vi "TestQTMCommander.vi"() -> ()   [LabVIEW 2017]
uses:
  Globals/QualisysInstruction.vi
panel:
  in  "StopCapture":bool
  in  "SendTrig":bool
  in  "stop":bool
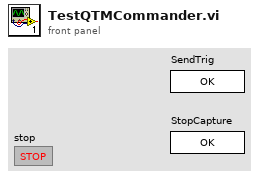
[diagram p1: front panel]
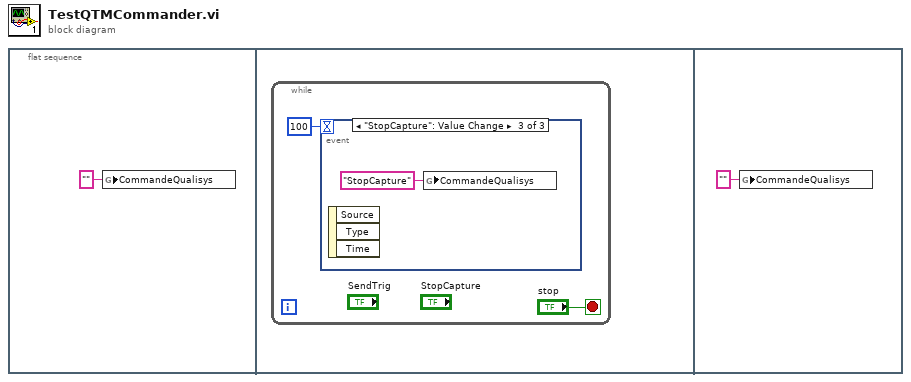
[diagram p0: block diagram]
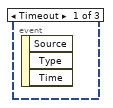
[diagram p2: hidden frame]
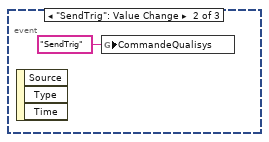
[diagram p3: hidden frame]
diagram:
  n1 = flat-sequence {
    frame #0 {
      n2 = global write "QualisysInstruction.vi" "CommandeQualisys"("" ("CommandeQualisys")) -> ()
    }
    frame #1 {
      n3 = while {
        stop <- "stop" stop-if-true
        n4 = event shown="[2] \"StopCapture\": Value Change" {
          selector: _ -> [_ _ _]
          dyn-events: _ -> [_ _ _]
          timeout: 100 -> [_ _ _]
          event Timeout {
            n5 = event-data() -> ()  [unwired: 1 in, 3 out]
          }
          event "SendTrig": Value Change {
            n6 = event-data() -> ()  [unwired: 1 in, 3 out]
            n7 = global write "QualisysInstruction.vi" "CommandeQualisys"("SendTrig" ("CommandeQualisys")) -> ()
          }
          event "StopCapture": Value Change {
            n8 = event-data() -> ()  [unwired: 1 in, 3 out]
            n9 = global write "QualisysInstruction.vi" "CommandeQualisys"("StopCapture" ("CommandeQualisys")) -> ()
          }
        }
      }
    }
    frame #2 {
      n10 = global write "QualisysInstruction.vi" "CommandeQualisys"("" ("CommandeQualisys")) -> ()
    }
  }
